vi "Example Typecast 1.vi"(8 "Error In":errorcluster) -> (0 "Error Out":errorcluster)   [LabVIEW 2014]
panel:
  out "*(type *) &x":string
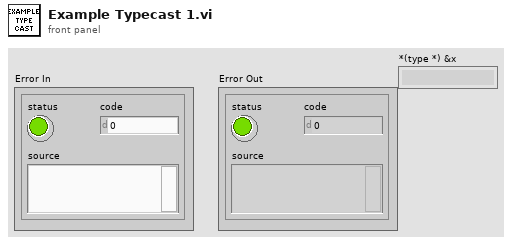
[diagram p1: front panel]
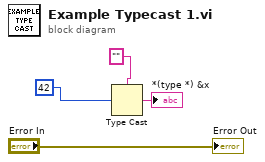
[diagram p0: block diagram]
diagram:
  n1 = Type Cast(type="", x=42) -> (*(type *) &x=→"*(type *) &x":string)
  "Error Out" <- "Error In"
